vi "Method No Arguments.vi"(8 "error in (no error)":errorcluster, 11 "Mock In":refnum<class "Test Interface Responsive Mock.lvclass">) -> (0 "error out":errorcluster, 3 "Mock Out":refnum<class "Test Interface Responsive Mock.lvclass">)   [LabVIEW 2020, in "Test Interface Responsive Mock.lvclass"]
uses:
  Test Interface Responsive Mock.lvclass
  C:/git/astemes-lmock/source/Framework/Mock/Mock.lvclass
  source/Framework/Mock/Mock.lvclass
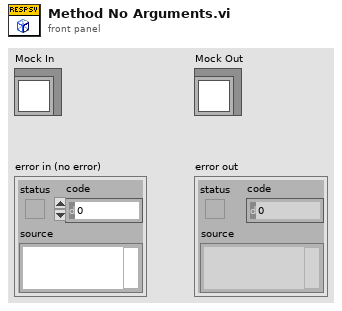
[diagram p1: front panel]
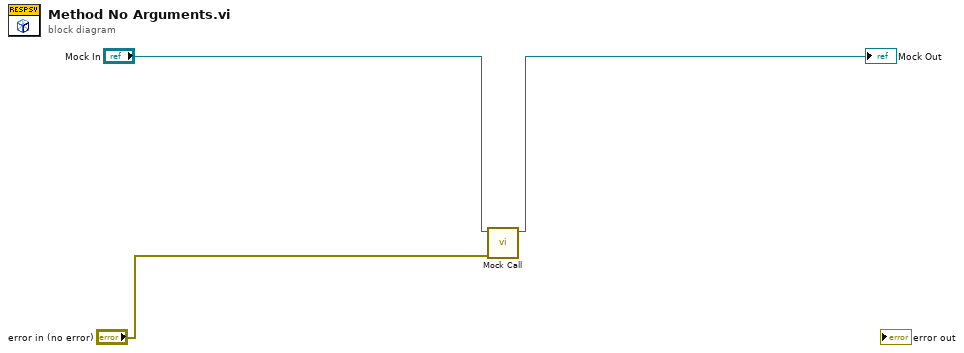
[diagram p0: block diagram]
diagram:
  n1 = call "Mock Call.vi"("error in (no error)"="error in (no error)", "Mock In"="Mock In") -> ("Mock Out"=→"Mock Out":refnum<class "Test Interface Responsive Mock.lvclass">)  [unwired: 8 in, 1 out]
